vi "Get Pattern Data.vi"(7 "theta":dbl, 8 "Iterative?":bool, 9 "File Name":i32[](array[numeric]), 10 "Folder Name":string, 11 "Dispense.lvclass":refnum<class "Dispense.lvclass">) -> (3 "Dispense Out":refnum<class "Dispense.lvclass">)   [LabVIEW 2019, in "Dispense.lvclass"]
uses:
  Dispense.lvclass
  Dispense.lvclass/Dispense.ctl
  <vilib>/Analysis/coordinate.llb/2D Cartesian Coordinate Rotation (Scalar).vi
  <vilib>/Analysis/NI_AALPro.lvlib
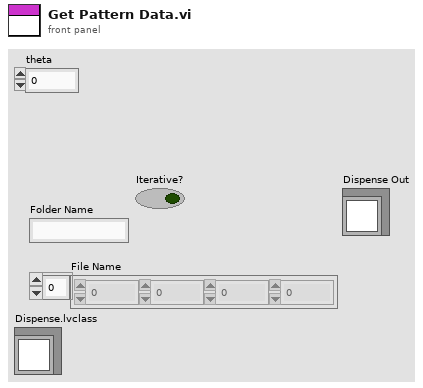
[diagram p1: front panel]
types:
  T1 = typedef "File Paths.ctl" = cluster{"Glue Pattern Folder":path, "Carrier Tray Folder":path, "Pick Up Tool Fixture Folder":path, "Components Folder":path, "Bellows Tool Offset.txt":path, "Pick Up Tool Offset.txt":path, "Dispense Tip Offset.txt":path, "Log Files":path}
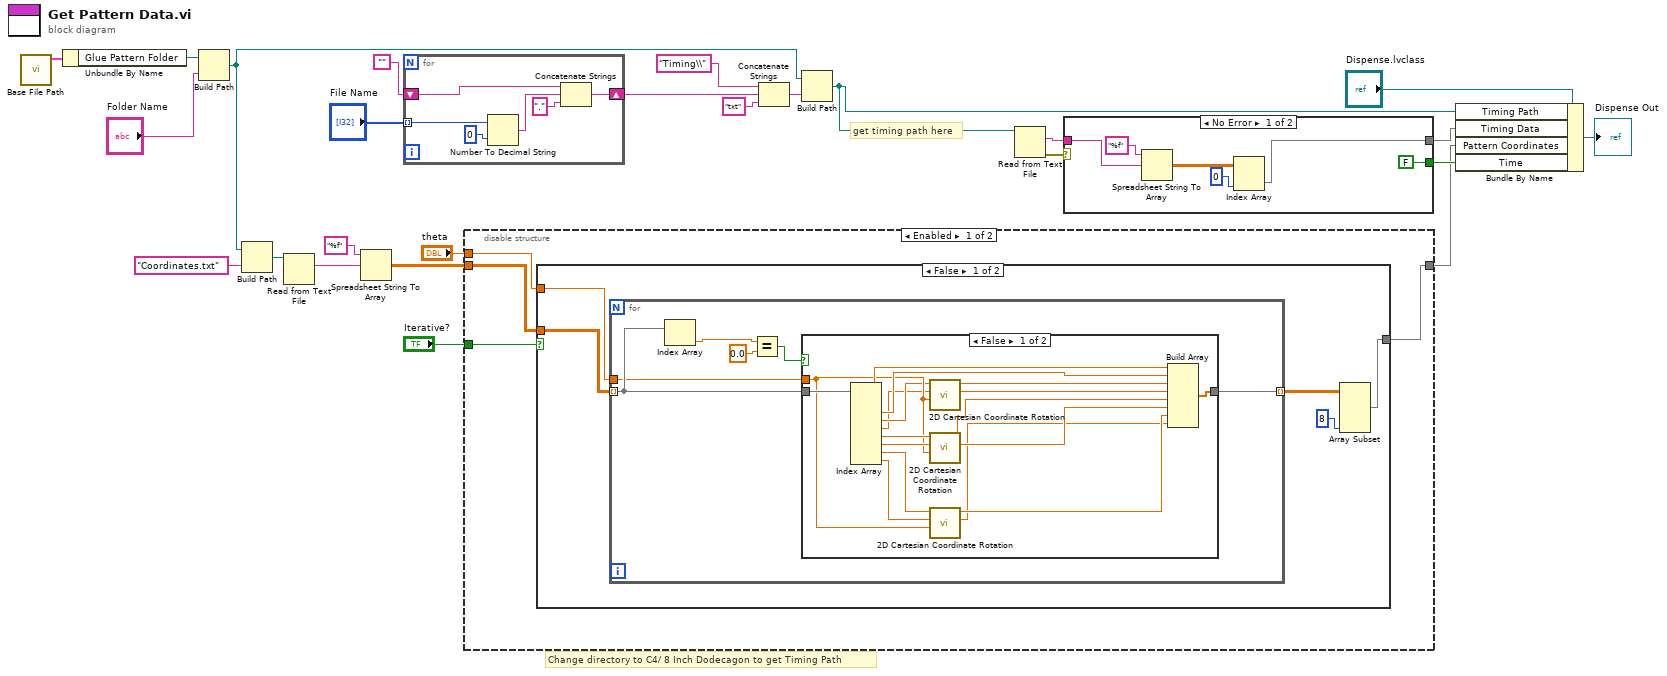
[diagram p0: block diagram]
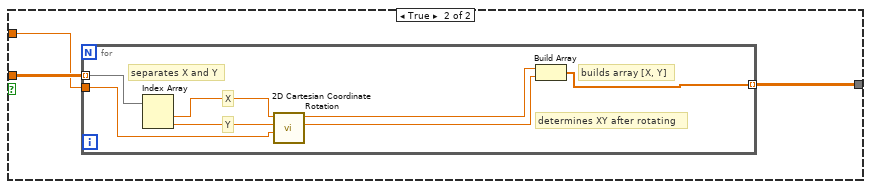
[diagram p3: hidden frame]
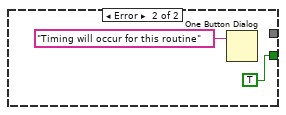
[diagram p5: hidden frame]
diagram:
  # "Change directory to C4/ 8 Inch Dodecagon to get Timing Path"
  # "get timing path here"
  n1 = call "Base File Path.vi"() -> ("Paths Out"=w12:T1)  [unwired: 11 in]
  n2 = Unbundle By Name(w12) -> ("Glue Pattern Folder"=w16:path)
  n3 = Build Path(base path=w16, name or relative path="Folder Name") -> (appended path=w23:path)
  n4 = Build Path(base path=w23, name or relative path="Coordinates.txt") -> (appended path=w18:path)
  n5 = Read from Text File(file (use dialog)=w18) -> (text=w14:string)  [unwired: 3 in, 3 out]
  n6 = Spreadsheet String To Array(format string="%f", spreadsheet string=w14) -> (array=w4:dbl[][])  [unwired: 2 in]
  n7 = for {
    tunnel: "File Name" -> [w31] mode=indexing
    shift-right: [w27] -> w21
    shift-left: "" -> [w26]
    n8 = Number To Decimal String(number=w31, width (-)=i16 0) -> (decimal integer string=w29:string)
    n9 = Concatenate Strings(w26, w29, "." ("string")) -> (w27:string)
  }
  n10 = disable-structure shown="Enabled" {
    disable-tunnel: "Iterative?" -> [w35 _]
    disable-tunnel: w4 -> [w34 w75]
    disable-tunnel: [w33 w75] -> w3
    disable-tunnel: "theta" -> [w32 _]
    frame Enabled {
      n11 = case shown="False" w35 {
        tunnel: w34 -> [w38 w67]
        tunnel: [w37 w66] -> w33
        tunnel: w32 -> [w36 w65]
        frame False {
          n12 = for {
            tunnel: w38 -> [w42] mode=indexing
            tunnel: [w43] -> w40 mode=indexing
            tunnel: w36 -> [w41]
            n13 = Index Array(array=w42) -> (element=w46:dbl)  [unwired: 1 in]
            n14 = Equal?(x=w46, y=0.0) -> (x = y?=w44:bool)
            n15 = case shown="False" w44 {
              tunnel: w42 -> [w63 w64]
              tunnel: [w62 w64] -> w43
              tunnel: w41 -> [w51 _]
              frame False {
                n16 = Index Array(array=w63) -> (element #1=w61:dbl, element #2=w60:dbl, element #3=w50:dbl, element #4=w49:dbl, element #5=w53:dbl, element #6=w52:dbl, element #7=w48:dbl, element #8=w47:dbl)  [unwired: 8 in]
                n17 = call-poly <vilib>:"2D Cartesian Coordinate Rotation.vi"("theta"=w51, "y"=w49, "x"=w50) -> ("y out"=w58:dbl, "x out"=w59:dbl)  [unwired: 6 in, 1 out]
                n18 = call-poly <vilib>:"2D Cartesian Coordinate Rotation.vi"("theta"=w51, "y"=w52, "x"=w53) -> ("y out"=w56:dbl, "x out"=w57:dbl)  [unwired: 6 in, 1 out]
                n19 = call-poly <vilib>:"2D Cartesian Coordinate Rotation.vi"("theta"=w51, "y"=w47, "x"=w48) -> ("y out"=w54:dbl, "x out"=w55:dbl)  [unwired: 6 in, 1 out]
                n20 = Build Array(w61, w60, w59, w58, w57, w56, w55, w54) -> (w62:dbl[])
              }
              frame True {
              }
            }
          }
          n21 = Array Subset(array=w40, length (col)=8 ("length")) -> (w37:dbl[][])  [unwired: 3 in]
        }
        frame True {
          n22 = for {
            tunnel: w67 -> [w74] mode=indexing
            tunnel: [w69] -> w66 mode=indexing
            tunnel: w65 -> [w68]
            # "separates X and Y"
            # "builds array [X, Y]"
            # "determines XY after rotating"
            # "Y"
            # "X"
            n23 = Index Array(array=w74) -> (element #1=w73:dbl, element #2=w72:dbl)  [unwired: 2 in]
            n24 = call-poly <vilib>:"2D Cartesian Coordinate Rotation.vi"("theta"=w68, "y"=w72, "x"=w73) -> ("y out"=w70:dbl, "x out"=w71:dbl)  [unwired: 6 in, 1 out]
            n25 = Build Array(w71, w70) -> (w69:dbl[])
          }
        }
      }
    }
    frame Disabled {
    }
  }
  n26 = Concatenate Strings("Timing\\" ("name or relative path"), w21, "txt" ("string")) -> (w24:string)
  n27 = Build Path(base path=w23, name or relative path=w24) -> (appended path=w10:path)
  n28 = Read from Text File(file (use dialog)=w10) -> (text=w25:string, error out=w5:errorcluster)  [unwired: 3 in, 2 out]
  n29 = case shown="No Error" w5 {
    tunnel: w25 -> [w80 _]
    tunnel: [w78 _] -> w9
    tunnel: [FALSE TRUE] -> w8
    frame No Error {
      n30 = Spreadsheet String To Array(format string="%f", spreadsheet string=w80) -> (array=w79:dbl[][])  [unwired: 2 in]
      n31 = Index Array(array=w79, index (col)=0 ("disabled index (col)")) -> (element=w78:dbl[])  [unwired: 1 in]
    }
    frame Error {
      n32 = One Button Dialog(message="Timing will occur for this routine") -> ()  [unwired: 1 in, 1 out]
    }
  }
  n33 = Bundle By Name(cluster="Dispense.lvclass", "Timing Path"=w10, "Timing Data"=w9, "Pattern Coordinates"=w3, "Time"=w8) -> (→"Dispense Out":refnum<class "Dispense.lvclass">)
